vi "Test Record Failing Method Result.vi"(8 "error in (no error)":errorcluster, 11 "Result Model Result Recording Test in":refnum<class "Result Model Result Recording Test.lvclass">) -> (0 "error out":errorcluster, 3 "Result Model Result Recording Test out":refnum<class "Result Model Result Recording Test.lvclass">)   [LabVIEW 2020, in "Result Model Result Recording Test.lvclass"]
uses:
  Result Model Result Recording Test.lvclass
  C:/Program Files (x86)/National Instruments/LabVIEW 2020/vi.lib/Astemes/LUnit/Test Case.lvclass
  Result/Result.ctl
  Result/Status.ctl
  Result/Type.ctl
  <vilib>/Astemes/LUnit/Test Case.lvclass/Test Case.ctl
  ae2c71b8-32bb-49d1-8500-0119bfec74ff.vi
  <vilib>/Astemes/LUnit/Palette/Pass.vi
  <vilib>/Astemes/LUnit/Palette/Fail.vi
  <vilib>/Astemes/LUnit/Compare Variants.vi
  <vilib>/Astemes/LUnit/Describe Comparison.vi
  <vilib>/Astemes/LUnit/Set Assertion Type.vi
  <vilib>/Astemes/LUnit/Add test result.vi
  <vilib>/Astemes/LUnit/Variant to string.vi
  <vilib>/Astemes/LUnit/LUnit Record Assertion Result.vi
  <vilib>/Astemes/LUnit/LUnit Aggregate Assertion Results.vi
  <vilib>/Astemes/LUnit/Method Result/LUnit Merge Status.vi
  <vilib>/Astemes/LUnit/LUnit Concatenate result strings.vi
  <vilib>/Utility/Data Type/Get Type Information.vi
  <vilib>/Utility/LVClass/Get LV Class Name.vi
  Result Model Result Recording Test.lvclass/Result Model Result Recording Test.ctl
  Result Model/Result Model.lvclass
  Result/Result.lvlib
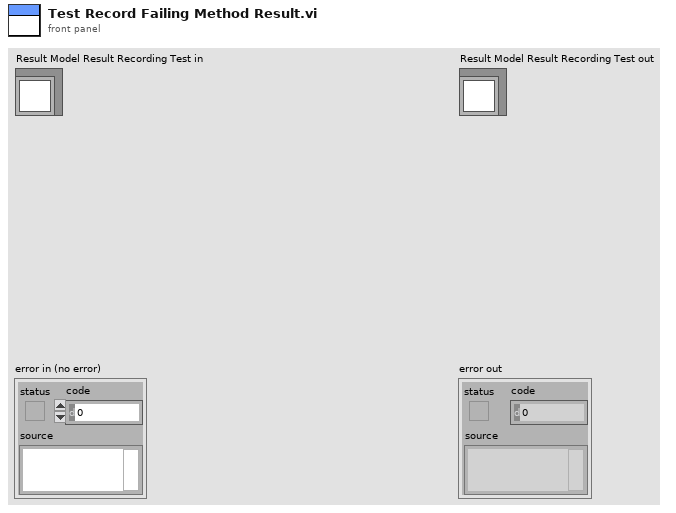
[diagram p1: front panel]
types:
  T1 = typedef "Result.lvlib/Result.ctl" = cluster{"Name":string, "Message":string, "Description":string, "Status":T2, "Result Type":T3, "Execution Time":dbl}
  T2 = typedef "Result.lvlib/Status.ctl" = enum16{"", "Passed", "Failed", "Error", "Skipped", "Setup Error", "Broken", "Teardown Error"}
  T3 = typedef "Result.lvlib/Type.ctl" = enum16{"Method", "Case", "Suite", "Pass", "Fail", "Skip", "Pass if", "Fail if", "Pass if Error", "Fail if Error", "Pass if Equal", "Fail if Equal"}
  T4 = cluster{"Left Cell String":string, "Child Text":string[], "Child Tag":string, "Item Indent":i32, "Child Only?":bool, "Glyph Index":i32}[]
  T5 = cluster{"Left Cell String":string, "Child Text":string[], "Child Tag":string, "Item Indent":i32, "Child Only?":bool, "Glyph Index":i32}
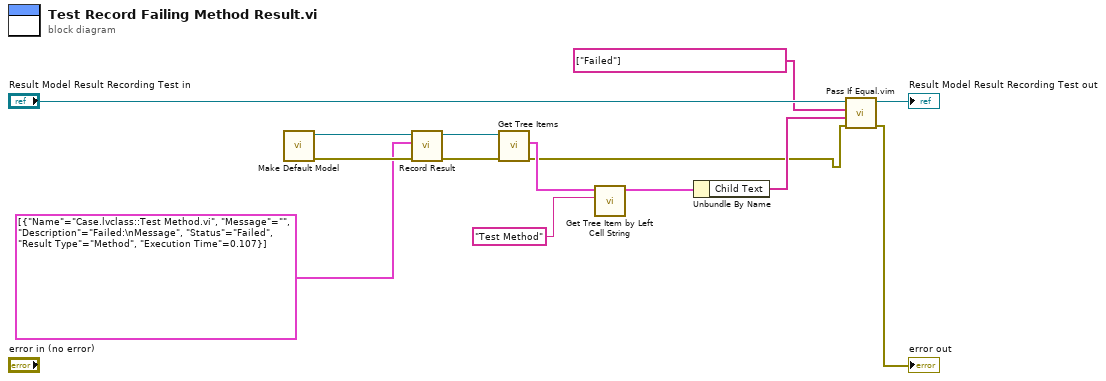
[diagram p0: block diagram]
diagram:
  n1 = call "Make Default Model.vi"() -> ("error out"=w13:errorcluster, "Result Model out"=w14:refnum<class "Result Model.lvclass">)  [unwired: 10 in]
  n2 = call "Record Result.vi"("error in (no error)"=w13, "Results"=T1[] [{"Name"="Case.lvclass::Test Method.vi", "Message"="", "Description"="Failed:\nMessage", "Status"=enum."Failed", "Result Type"=enum."Method", "Execution Time"=0.107}], "Result Model in"=w14) -> ("error out"=w10:errorcluster, "Result Model out"=w11:refnum<class "Result Model.lvclass">)  [unwired: 7 in]
  n3 = call "Get Tree Items.vi"("error in (no error)"=w10, "Result Model In"=w11) -> ("error out"=w1:errorcluster, "Tree Items"=w9:T4)  [unwired: 7 in, 1 out]
  n4 = call "Get Tree Item by Left Cell String.vi"("Left Cell String"="Test Method", "Tree Items"=w9) -> ("Item"=w5:T5)  [unwired: 9 in]
  n5 = Unbundle By Name(w5) -> ("Child Text"=w4:string[])
  n6 = call "Pass If Equal.vim"("error in (no error)"=w1, "Actual"=w4, "Expected"=string[] ["Failed"] ("Child Text"), "LUnit Test Case In"="Result Model Result Recording Test in") -> ("error out"=→"error out":errorcluster, "LUnit Test Case Out"=→"Result Model Result Recording Test out":refnum<class "Result Model Result Recording Test.lvclass">)  [unwired: 6 in]
